vi "create.vi"(8 "error in (no error)":errorcluster, 10 "handle":i32, 11 "client":i32) -> (0 "error out":errorcluster, 3 "AssetCreateStaging out":refnum<class "AssetCreateStaging.lvclass">)   [LabVIEW 2020, in "AssetCreateStaging.lvclass"]
uses:
  AssetCreateStaging.lvclass
  AssetCreateStaging.lvclass/AssetCreateStaging.ctl
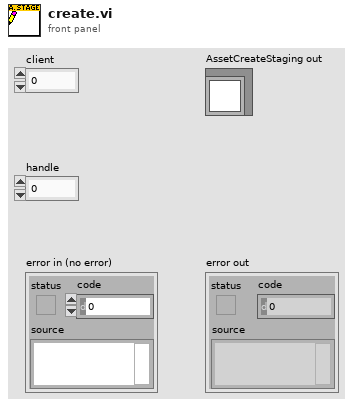
[diagram p1: front panel]
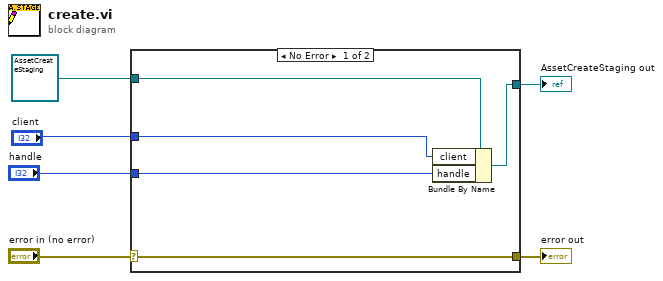
[diagram p0: block diagram]
diagram:
  n1 = case shown="No Error" "error in (no error)" {
    selector: "error in (no error)" -> [w11 w12]
    tunnel: [w11 w12] -> w5
    tunnel: [w9 w13] -> w3
    tunnel: refnum<class "AssetCreateStaging.lvclass"> refnum ("AssetCreateStaging in") -> [w10 w13]
    tunnel: "handle" -> [w8 _]
    tunnel: "client" -> [w7 _]
    frame No Error {
      n2 = Bundle By Name(cluster=w10, "client"=w7, "handle"=w8) -> (w9:refnum<class "AssetCreateStaging.lvclass">)
    }
    frame Error {
    }
  }
  "error out" <- w5
  "AssetCreateStaging out" <- w3
